vi "testShutdown.vi"   [LabVIEW 2014]
types:
  T1 = enum16{"Left Button", "Center Button", "Right Button", "Window Close"}
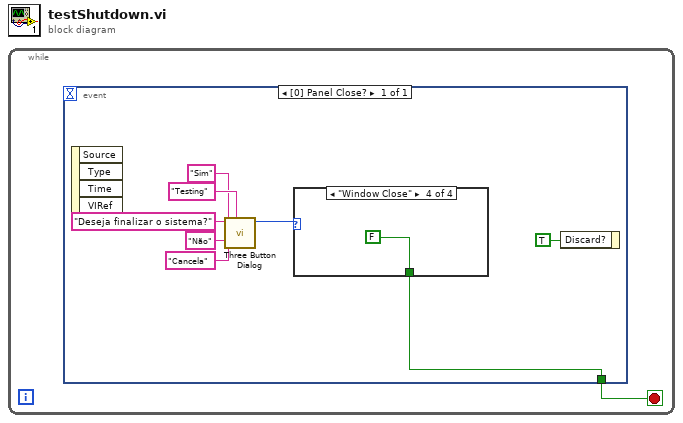
[diagram p0: block diagram]
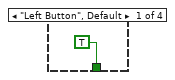
[diagram p2: hidden frame]
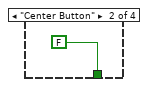
[diagram p3: hidden frame]
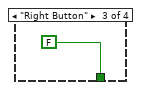
[diagram p4: hidden frame]
diagram:
  n1 = while {
    stop <- w1 stop-if-true
    n2 = event shown="[0] Panel Close?" {
      selector: _ -> [_]
      dyn-events: _ -> [_]
      timeout: _ -> [_]
      tunnel: [w2] -> w1
      event Panel Close? {
        n3 = event-data() -> ()  [unwired: 1 in, 4 out]
        n4 = call <vilib>:"Three Button Dialog.vi"("Window Title (\"\")"="Testing" ("Window Title (\"\")"), "Right Button Text (\"Cancel\")"="Cancela" ("Right Button Text (\"Cancel\")"), "Center Button Text (\"No\")"="Não" ("Center Button Text (\"No\")"), "Left Button Text (\"Yes\")"="Sim" ("Left Button Text (\"Yes\")"), "message"="Deseja finalizar o sistema?") -> ("Which Button?"=w8:T1)  [unwired: 6 in]
        n5 = case shown="\"Window Close\"" w8 {
          tunnel: [TRUE FALSE FALSE FALSE] -> w2
          frame "Left Button", Default {
          }
          frame "Center Button" {
          }
          frame "Right Button" {
          }
          frame "Window Close" {
          }
        }
        n6 = event-data("Discard?"=TRUE) -> ()  [unwired: 1 in, 1 out]
      }
    }
  }
